vi "Example Simple Voltage.vi"() -> ()   [LabVIEW 2013]
uses:
  C:/tf/play/labview/Tinkerforge.dll
  Tinkerforge.dll
panel:
  in  "uid":string="amb"
  in  "port":i32=4223
  in  "host":string="localhost"
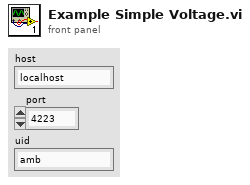
[diagram p1: front panel]
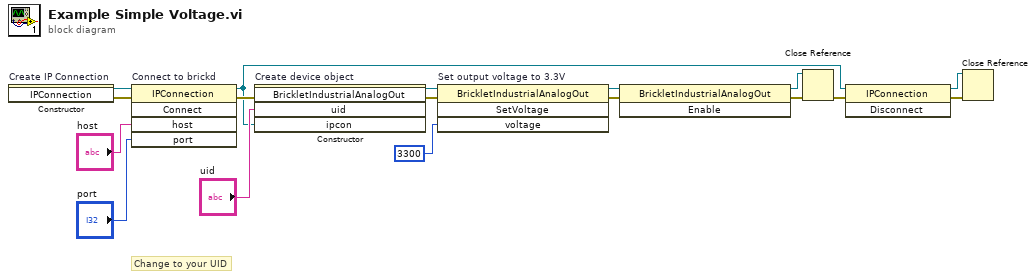
[diagram p0: block diagram]
diagram:
  # "Change to your UID"
  n1 = constructor on="Create IP Connection" class="IPConnection"() -> (reference out=w17:refnum<k24>, error out=w5:errorcluster)  [unwired: 3 in, 1 out]
  n2 = invoke on="Connect to brickd" class="IPConnection" method="Connect"(reference=w17, error in=w5, "host"="host", "port"="port") -> (reference out=w8:refnum<k24>, error out=w13:errorcluster)  [unwired: 1 in, 3 out]
  n3 = constructor on="Create device object" class="BrickletIndustrialAnalogOut"(error in=w13, "uid"="uid", "ipcon"=w8) -> (reference out=w11:refnum<k24>, error out=w12:errorcluster)  [unwired: 2 in, 3 out]
  n4 = invoke on="Set output voltage to 3.3V" class="BrickletIndustrialAnalogOut" method="SetVoltage"(reference=w11, error in=w12, "voltage"=3300) -> (reference out=w2:refnum<k24>, error out=w4:errorcluster)  [unwired: 1 in, 2 out]
  n5 = invoke class="BrickletIndustrialAnalogOut" method="Enable"(reference=w2, error in=w4) -> (reference out=w1:refnum<k24>, error out=w3:errorcluster)  [unwired: 1 in, 1 out]
  n6 = Close Reference(reference=w1, error in (no error)=w3) -> (error out=w10:errorcluster)
  n7 = invoke class="IPConnection" method="Disconnect"(reference=w8, error in=w10) -> (reference out=w7:refnum<k24>, error out=w9:errorcluster)  [unwired: 1 in, 1 out]
  n8 = Close Reference(reference=w7, error in (no error)=w9) -> ()  [unwired: 1 out]
